vi "24G_FMCW_range.vi"() -> ()   [LabVIEW 2015]
doc: "This example demonstrates how to use the Short-time Fourier Transform (STFT Spectrograms) VI to analyze the Time-Frequency spectrogram."
uses:
  <vilib>/Analysis/baseanly.llb/Mean (DBL).vi
  <vilib>/Analysis/2dsp.llb/Real FFT.vi
  <vilib>/sound2/lvsound2.llb/Sound Input Read (DBL).vi
  <vilib>/Analysis/NI_AALPro.lvlib
  <vilib>/Analysis/NI_AALBase.lvlib
  <vilib>/Analysis/NI_AAL_SigProc.lvlib
panel:
  out "distance mm":dbl
  out "peak location":dbl
  in  "peak threshold":dbl=0.95 format="%0.2f"
  in  "duty ratio":dbl=0.6
  out "Spectrum":waveform(dbl)(graph)
  in  "begin offsets":i32=10
  in  "end offsets":i32
  out "max range":dbl
  out "range resolution":dbl
  out "chirp rate":dbl
  out "real time chirp frequency":dbl
  in  "FFT length":i32=4096
  in  "slow-time frequency":dbl=417.0
  out "average samples per chirp":i32
  in  "threshold":dbl=0.6 format="%0.2f"
  in  "bits per sample":i32=16
  in  "number of channels":i32=2
  in  "sample rate (S/s)":dbl=192000.0
  in  "number of samples/ch":i32=40000 min=1024 max=100000
  in  "Numeric Control":dbl=1.0
  in  "device ID":u32
  in  "Stop":bool
  # "FMCW Radar Realtime Range Detection"
  # "Version: 1\nZhengyu Peng\nC. Li Lab\nTexas Tech University\nFeb. 2016"
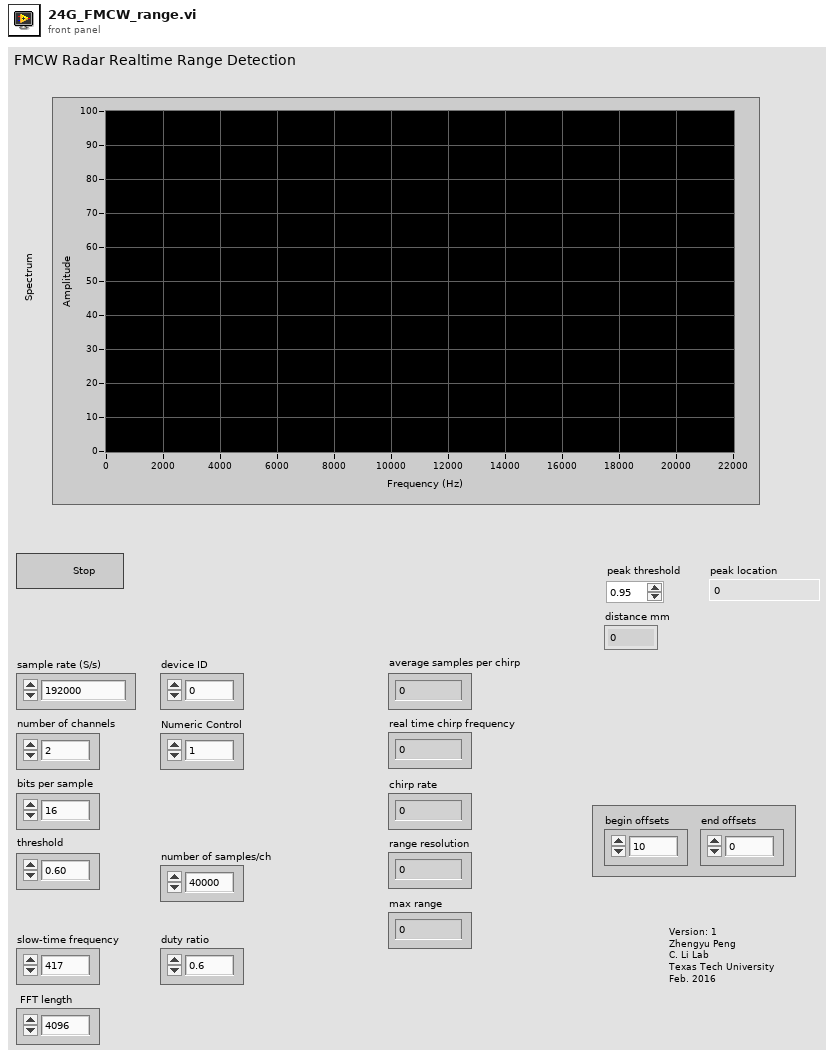
[diagram p1: front panel]
types:
  T1 = cluster{"sample rate (S/s)":dbl, "number of channels":i32, "bits per sample ":i32}
  T2 = typedef "Sound Input Task ID.ctl" = u32
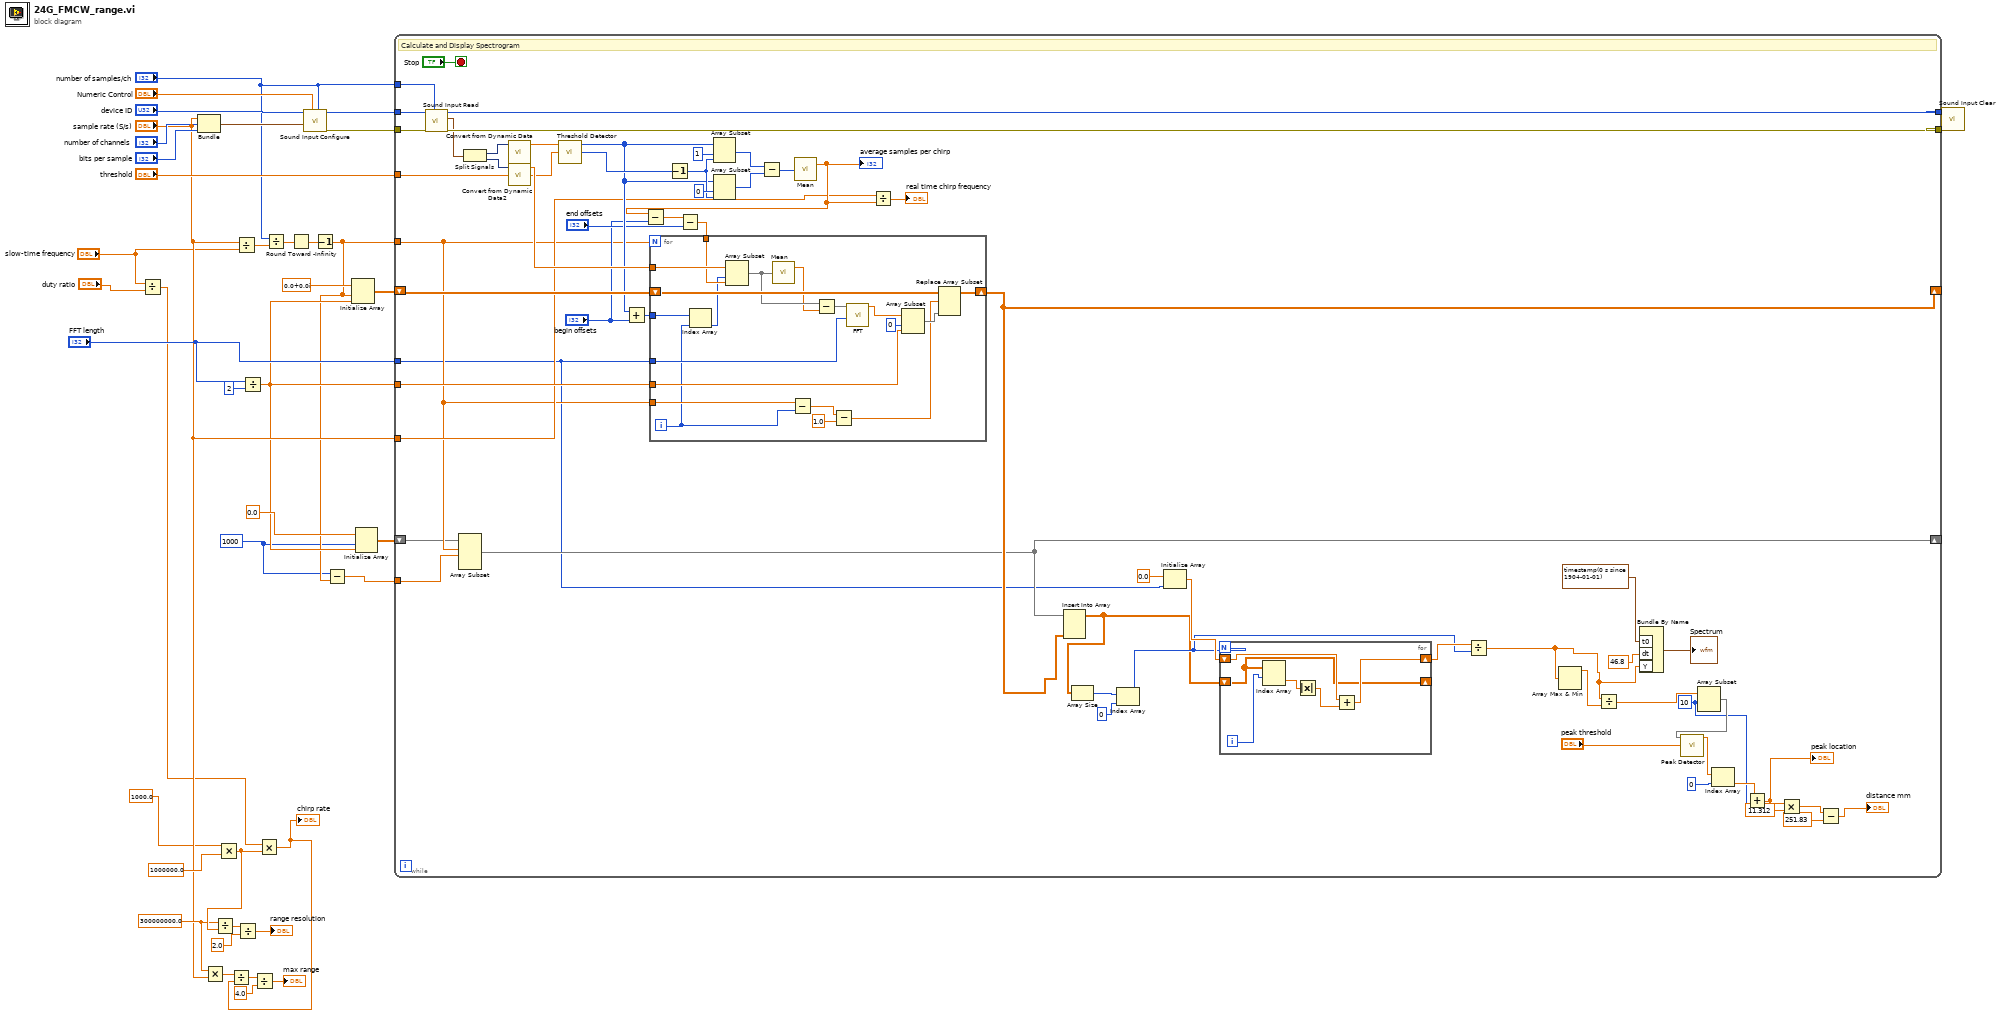
[diagram p0: block diagram]
diagram:
  w3 = 1000 ("dimension size")
  w18 = 300000000.0 ("x")
  n1 = Divide(x="slow-time frequency", y="duty ratio") -> (x/y=w9:dbl)
  n2 = Bundle("sample rate (S/s)"="sample rate (S/s)", "number of channels"="number of channels", "bits per sample"="bits per sample") -> (w30:T1)  [unwired: 1 in]
  n3 = Multiply(x=w18, y="sample rate (S/s)") -> (x*y=w17:dbl)
  n4 = Multiply(x=1000.0, y=1000000.0) -> (x*y=w22:dbl)
  n5 = Divide(x=w18, y=w22) -> (x/y=w21:dbl)
  n6 = Divide(x="sample rate (S/s)", y="slow-time frequency") -> (x/y=w26:dbl)
  n7 = Divide(x=w21, y=2.0) -> (x/y=→"range resolution":dbl)
  n8 = Divide(x="FFT length", y=2) -> (x/y=w6:dbl)
  n9 = Multiply(x=w9, y=w22) -> (x*y=w16:dbl)
  "chirp rate" <- w16
  n10 = Divide(x=w17, y=w16) -> (x/y=w15:dbl)
  n11 = Divide(x=w15, y=4.0) -> (x/y=→"max range":dbl)
  n12 = Divide(x="number of samples/ch", y=w26) -> (x/y=w25:dbl)
  n13 = Round Toward -Infinity(1:w25) -> (0:w24:dbl)
  n14 = call <vilib>:"Sound Input Configure.vi"("number of samples/ch"="number of samples/ch", "sample mode"="Numeric Control", "sound format"=w30, "device ID"="device ID") -> ("error out"=w37:errorcluster, "task ID"=w39:T2)  [unwired: 6 in]
  n15 = Decrement(x=w24) -> (x-1=w5:dbl)
  n16 = Subtract(x=w3, y=w5) -> (x-y=w4:dbl)
  n17 = Initialize Array(cdb 0.0+0.0i ("element"), w5, w6) -> (w28:cdb[][])
  n18 = Initialize Array(0.0 ("element"), w3, w6) -> (w33:dbl[][])
  n19 = while {
    tunnel: w39 -> [w99]
    tunnel: "number of samples/ch" -> [w98]
    tunnel: w37 -> [w97]
    tunnel: [w96] -> w36
    tunnel: [w95] -> w35
    shift-right: [w57] -> _
    shift-left: w33 -> [w58]
    shift-right: [w59] -> _
    shift-left: w28 -> [w83]
    tunnel: "threshold" -> [w81]
    tunnel: w5 -> [w61]
    tunnel: "sample rate (S/s)" -> [w71]
    tunnel: "FFT length" -> [w54]
    tunnel: w6 -> [w79]
    tunnel: w4 -> [w55]
    stop <- "Stop" stop-if-true
    w48 = 10 ("index")
    # "Calculate and Display Spectrogram"
    n20 = call-poly <vilib>:"Sound Input Read.vi"("number of samples/ch"=w98, "error in (no error)"=w97, "task ID"=w99) -> ("error out"=w95:errorcluster, "data"=w92:waveform(dbl)[], "task ID out"=w96:T2)  [unwired: 6 in]
    n21 = Array Subset(array=w58, index (row)=w61, length (row)=w55) -> (w57:dbl[][])  [unwired: 2 in]
    n22 = Split Signals(w92) -> (w94:dynamicdata, w93:dynamicdata)  [unwired: 2 out]
    n23 = call "Convert from Dynamic Data"("Dynamic Data Type"=w94) -> ("Array"=w91:dbl[])  [unwired: 3 out]
    n24 = call "Convert from Dynamic Data2"("Dynamic Data Type"=w93) -> ("Array"=w82:dbl[])  [unwired: 3 out]
    n25 = call <vilib>:"Threshold Detector.vi"("threshold"=w81, "X"=w91) -> ("count"=w86:i32, "Indices"=w78:i32[])  [unwired: 1 in, 1 out]
    n26 = Add(x=w78, y="begin offsets") -> (x+y=w77:i32[])
    n27 = Decrement(x=w86) -> (x-1=w85:i32)
    n28 = Array Subset(array=w78, index=1, length=w85) -> (w88:i32[])
    n29 = Array Subset(array=w78, index=0, length=w85) -> (w87:i32[])
    n30 = Subtract(x=w88, y=w87) -> (x-y=w84:i32[])
    n31 = call-poly <vilib>:"Mean.vi"("X"=w84) -> ("mean"=w74:dbl)  [unwired: 1 out]
    "average samples per chirp" <- w74
    n32 = Subtract(x=w74, y="begin offsets") -> (x-y=w72:dbl)
    n33 = Subtract(x=w72, y="end offsets") -> (x-y=w76:dbl)
    n34 = for {
      N: w61 -> [_]
      tunnel: w82 -> [w124]
      tunnel: w76 -> [w123]
      tunnel: w77 -> [w122]
      shift-right: [w120] -> w59
      shift-left: w83 -> [w125]
      tunnel: w54 -> [w113]
      tunnel: w79 -> [w115]
      tunnel: w61 -> [w112]
      i -> [w111]
      n35 = Index Array(array=w122, index=w111) -> (element=w121:i32)
      n36 = Array Subset(array=w124, index=w121, length=w123) -> (w119:dbl[])
      n37 = call-poly <vilib>:"Mean.vi"("X"=w119) -> ("mean"=w118:dbl)  [unwired: 1 out]
      n38 = Subtract(x=w112, y=w111) -> (x-y=w109:dbl)
      n39 = Subtract(x=w119, y=w118) -> (x-y=w117:dbl[])
      n40 = Subtract(x=w109, y=1.0) -> (x-y=w107:dbl)
      n41 = call-poly <vilib>:"FFT.vi"("FFT size"=w113, "X"=w117) -> ("FFT {X}"=w114:cdb[])  [unwired: 8 in, 1 out]
      n42 = Array Subset(array=w114, index=0, length=w115) -> (w110:cdb[])
      n43 = Replace Array Subset(array=w125, new element=w110, index (row)=w107) -> (w120:cdb[][])  [unwired: 1 in]
    }
    n44 = Divide(x=w71, y=w74) -> (x/y=→"real time chirp frequency":dbl)
    n45 = Insert Into Array(array=w57, new element=w59) -> (w60:dbl[][])  [unwired: 2 in]
    n46 = Array Size(array=w60) -> (size(s)=w70:i32[])
    n47 = Index Array(array=w70, index=0) -> (element=w65:i32)
    n48 = Initialize Array(0.0 ("element"), w54) -> (w67:dbl[])
    n49 = for {
      N: w65 -> [_]
      shift-right: [w103] -> _
      shift-left: w60 -> [w103]
      shift-right: [w105] -> w66
      shift-left: w67 -> [w106]
      i -> [w104]
      n50 = Index Array(array=w103, index (row)=w104) -> (element=w101:dbl[])  [unwired: 1 in]
      n51 = Absolute Value(x=w101) -> (abs(x)=w102:dbl[])
      n52 = Add(x=w106, y=w102) -> (x+y=w105:dbl[])
    }
    n53 = Divide(x=w66, y=w65) -> (x/y=w42:dbl[])
    n54 = Array Max & Min(array=w42) -> (max value=w56:dbl)  [unwired: 3 out]
    n55 = Divide(x=w42, y=w56) -> (x/y=w41:dbl[])
    n56 = Bundle By Name("t0"=timestamp(0 s since 1904-01-01), "dt"=46.8, "Y"=w42) -> (→"Spectrum":waveform(dbl))  [unwired: 1 out]
    n57 = Array Subset(array=w41, index=w48) -> (w50:dbl[])  [unwired: 1 in]
    n58 = call <vilib>:"Peak Detector.vi"("threshold"="peak threshold", "X"=w50) -> ("Locations"=w51:dbl[])  [unwired: 5 in, 4 out]
    n59 = Index Array(array=w51, index=0) -> (element=w49:dbl)
    n60 = Add(x=w49, y=w48) -> (x+y=w47:dbl)
    "peak location" <- w47
    n61 = Multiply(x=w47, y=11.312) -> (x*y=w45:dbl)
    n62 = Subtract(x=w45, y=251.83) -> (x-y=→"distance mm":dbl)
  }
  n63 = call <vilib>:"Sound Input Clear.vi"("error in (no error)"=w35, "task ID"=w36) -> ()  [unwired: 9 in, 1 out]
